vi "handleRecord.vi"(8 "error in (no error)":errorcluster, 10 "Record":refnum<class "Record.lvclass">, 11 "Handler.UserEvent in":refnum<class "Handler.UserEvent.lvclass">) -> (0 "error out":errorcluster, 3 "Handler.UserEvent out":refnum<class "Handler.UserEvent.lvclass">)   [LabVIEW 2017, in "Error Log.lvlib" / "Handler.UserEvent.lvclass"]
uses:
  Handler.UserEvent.lvclass
  Record/Record.lvclass
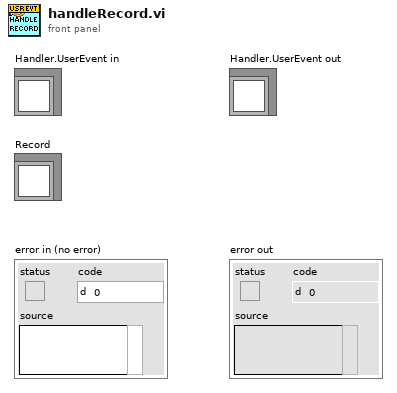
[diagram p1: front panel]
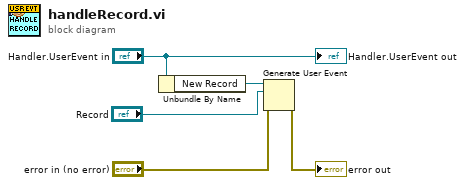
[diagram p0: block diagram]
diagram:
  n1 = Unbundle By Name("Handler.UserEvent in") -> ("New Record"=w4:refnum<user-event>)
  n2 = Generate User Event(user event=w4, event data cluster="Record", error in="error in (no error)") -> (error out=→"error out":errorcluster)  [unwired: 1 in, 1 out]
  "Handler.UserEvent out" <- "Handler.UserEvent in"
